vi "stream_data.vi"(7 "timeout in ms (-1)":i32, 8 "error in (no error)":errorcluster, 9 "Display":refnum<notifier>, 10 "Response":refnum<notifier>, 11 "Command":refnum<notifier>) -> (0 "error out":errorcluster)   [LabVIEW 2016]
uses:
  controls/Sensor_Data.ctl
  controls/MAG_UI_Command.ctl
  controls/MAG_Comms_State.ctl
panel:
  out "response":string
  in  "Update Delay (dT)":i32(slide)=100 scale=20.0..100.0
  out "Streaming Data IO":bool
  in  "Stop Button":bool
  out "dT":i32
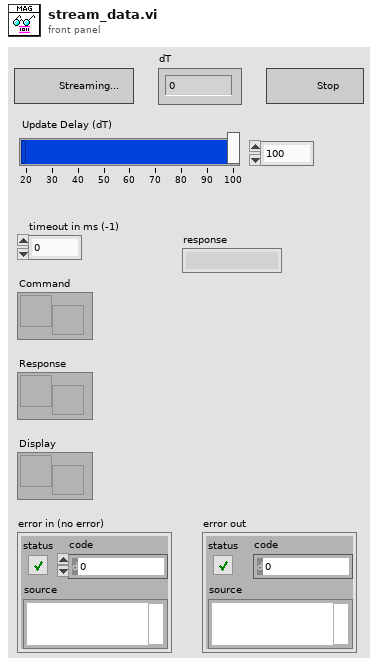
[diagram p1: front panel]
types:
  T1 = typedef "Sensor_Data.ctl" = cluster{"Time":u32, "Data":i16[]}
  T2 = typedef "MAG_UI_Command.ctl" = cluster{"Comms_States":T3, "Parameters":string, "Clear Buffer?":bool}
  T3 = typedef "MAG_Comms_State.ctl" = enum16{"Initialize", "Wait for Event", "Connect", "Send_Com", "Rcv_TXT", "Rcv_BIN", "Rcv_FILE", "Disconnect"}
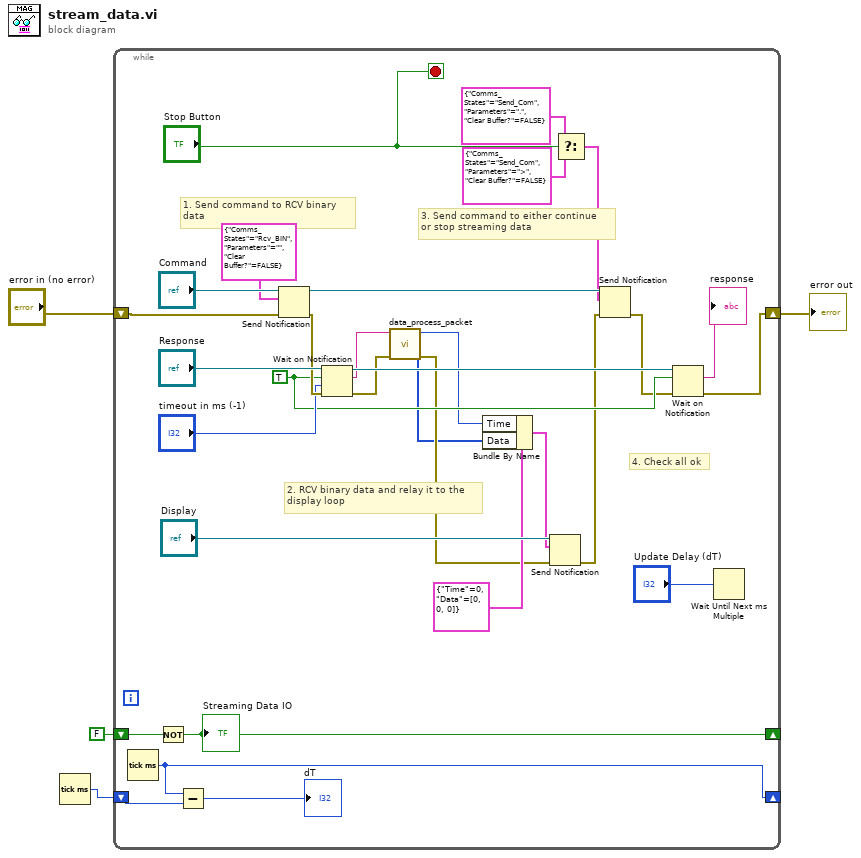
[diagram p0: block diagram]
diagram:
  n1 = Tick Count (ms)() -> (millisecond timer value=w1:u32)
  n2 = while {
    shift-right: [w19] -> w3
    shift-left: "error in (no error)" -> [w20]
    shift-right: [w16] -> _
    shift-left: FALSE -> [w17]
    shift-right: [w6] -> _
    shift-left: w1 -> [w8]
    stop <- "Stop Button" stop-if-true
    w24 = TRUE ("ignore previous (F)")
    # "4. Check all ok"
    # "3. Send command to either continue\nor stop streaming data"
    # "2. RCV binary data and relay it to the \ndisplay loop"
    # "1. Send command to RCV binary\ndata"
    n3 = Tick Count (ms)() -> (millisecond timer value=w6:u32)
    n4 = Not(x=w17) -> (.not. x?=w16:bool)
    "Streaming Data IO" <- w16
    n5 = Subtract(x=w6, y=w8) -> (x-y=→"dT":u32)
    n6 = Send Notification(notification=T2 {"Comms_States"=enum."Rcv_BIN", "Parameters"="", "Clear Buffer?"=FALSE}, notifier="Command", error in (no error)=w20) -> (notifier out=w29:refnum<notifier>, error out=w33:errorcluster)
    n7 = Wait on Notification(notifier="Response", ignore previous (F)=w24, timeout in ms (-1)="timeout in ms (-1)", error in (no error)=w33) -> (notifier out=w25:refnum<notifier>, notification=w15:string, error out=w14:errorcluster)  [unwired: 1 out]
    n8 = call "data_process_packet.vi"("error in (no error)"=w14, "Data Packet"=w15) -> ("error out"=w13:errorcluster, "Sensor Readings (Signed)"=w10:i16[], "Time"=w12:u32)  [unwired: 6 in, 1 out]
    n9 = Bundle By Name(cluster=T1 {"Time"=0, "Data"=[0, 0, 0]} ("notification"), "Time"=w12, "Data"=w10) -> (w9:T1)
    n10 = Send Notification(notification=w9, notifier="Display", error in (no error)=w13) -> (error out=w23:errorcluster)  [unwired: 1 out]
    n11 = Select(t=T2 {"Comms_States"=enum."Send_Com", "Parameters"=".", "Clear Buffer?"=FALSE}, s="Stop Button", f=T2 {"Comms_States"=enum."Send_Com", "Parameters"=">", "Clear Buffer?"=FALSE}) -> (s? t:f=w26:T2)
    n12 = Send Notification(notification=w26, notifier=w29, error in (no error)=w23) -> (error out=w22:errorcluster)  [unwired: 1 out]
    n13 = Wait on Notification(notifier=w25, ignore previous (F)=w24, error in (no error)=w22) -> (notification=→"response":string, error out=w19:errorcluster)  [unwired: 1 in, 2 out]
    n14 = Wait Until Next ms Multiple(millisecond multiple="Update Delay (dT)") -> ()  [unwired: 1 out]
  }
  "error out" <- w3
